vi "Calibrate XBox Controller.vi"() -> ()   [LabVIEW 2011]
panel:
  out "element":T1
  in  "Set Device Index":i32
  out "Steer Axis":i32
  out "Drive Axis":i32
  out "Stop":bool
  out "Joystick ID":refnum<k1>
  in  "stop":bool
  out "Acquire Error":errorcluster
  out "Initialize Error":errorcluster
  out "Close Error":errorcluster
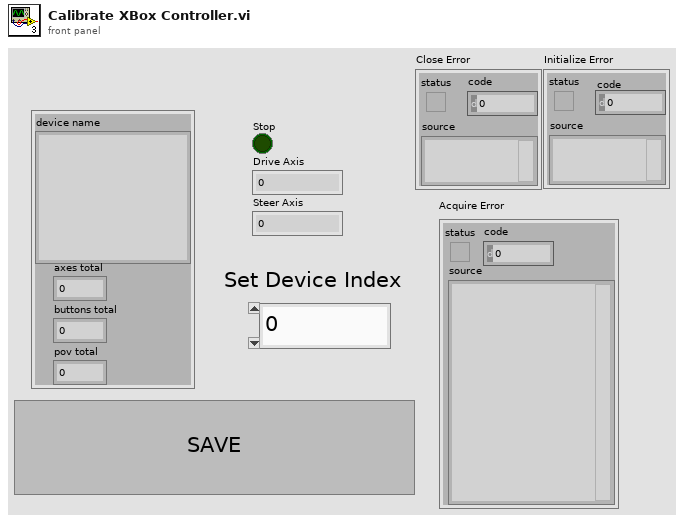
[diagram p1: front panel]
types:
  T1 = cluster{"axes total":u32, "buttons total":u32, "pov total":u32, "device name":string}
  T2 = cluster{"axes total":u32, "buttons total":u32, "pov total":u32, "device name":string}[]
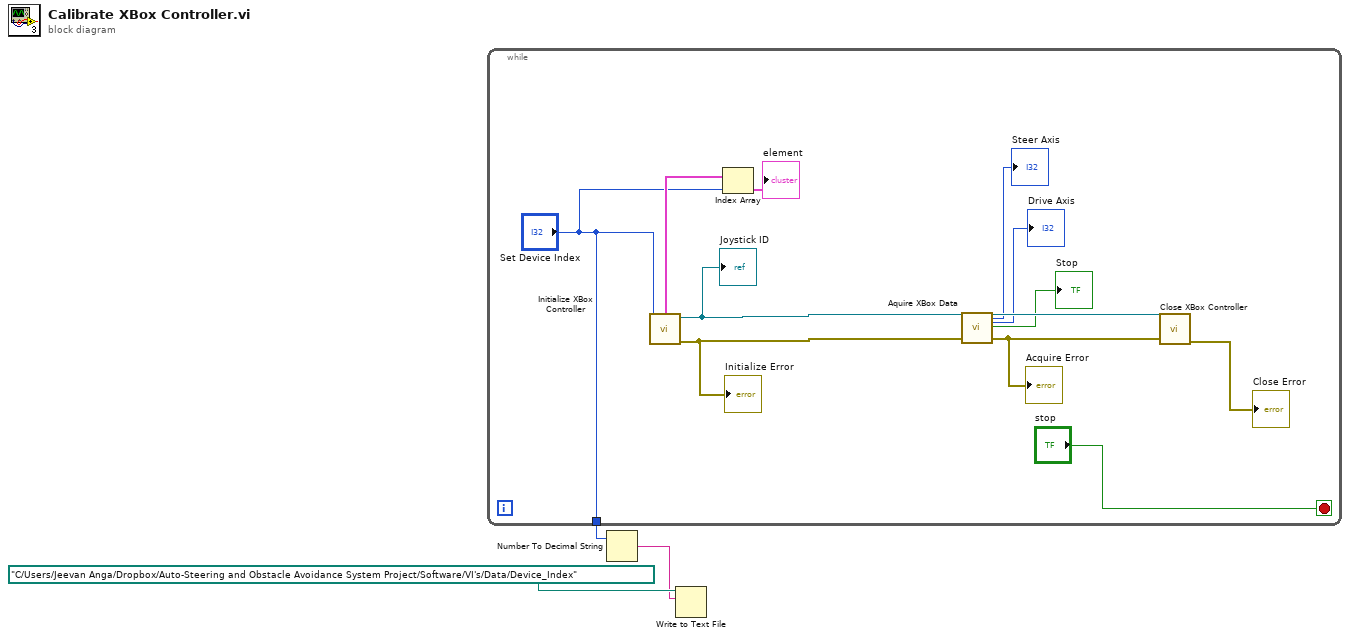
[diagram p0: block diagram]
diagram:
  n1 = while {
    tunnel: ["Set Device Index"] -> w2
    stop <- "stop" stop-if-true
    n2 = call "Initialize XBox Controller.vi"("XBox Device Index"="Set Device Index") -> ("error out"=w14:errorcluster, "device ID"=w15:refnum<k1>, "joystick info"=w6:T2)  [unwired: 8 in]
    "Initialize Error" <- w14
    "Joystick ID" <- w15
    n3 = Index Array(array=w6, index="Set Device Index") -> (element=→"element":T1)
    n4 = call "Aquire XBox Data.vi"("device ID"=w15, "error in (no error)"=w14) -> ("device ID 2"=w11:refnum<k1>, "Steer Axis"=→"Steer Axis":i32, "Drive Axis"=→"Drive Axis":i32, "Stop"=→"Stop":bool, "error out"=w12:errorcluster)  [unwired: 19 in, 2 out]
    "Acquire Error" <- w12
    n5 = call "Close XBox Controller.vi"("error in (no error)"=w12, "device ID"=w11) -> ("error out"=→"Close Error":errorcluster)  [unwired: 9 in]
  }
  n6 = Number To Decimal String(number=w2) -> (decimal integer string=w1:string)  [unwired: 1 in]
  n7 = Write to Text File(file (use dialog)=path "C:/Users/Jeevan Anga/Dropbox/Auto-Steering and Obstacle Avoidance System Project/Software/VI's/Data/Device_Index", text=w1) -> ()  [unwired: 2 in, 3 out]
